vi "W9EO82,FBO8PP_1,.vi"() -> ()   [LabVIEW 2023]
panel:
  out "Gauge":dbl[unit](knob)
  out "Eredmény":dbl[unit]
  in  "Bevitel":dbl[unit]
  in  "Gomb":bool
  out "Led":bool
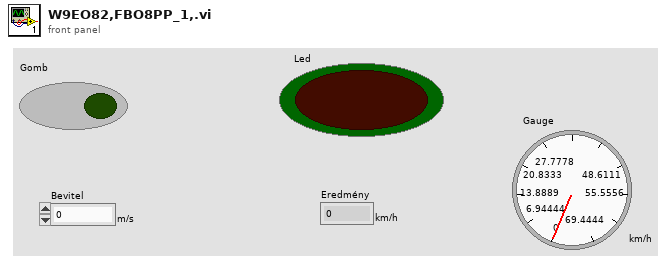
[diagram p1: front panel]
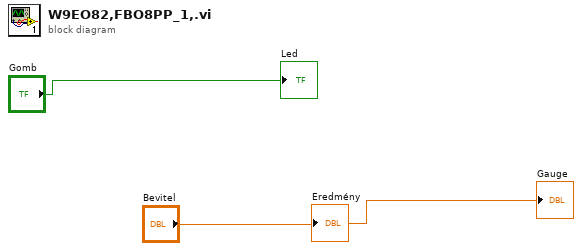
[diagram p0: block diagram]
diagram:
  "Led" <- "Gomb"
  "Eredmény" <- "Bevitel"
  "Gauge" <- "Bevitel"
